vi "serialization tests.vi"() -> ()   [LabVIEW 2013, in "Modbus Slave tests.lvlib"]
doc: "Platypus Framework 1.0.1.65\nNI Systems Engineering - National Instruments"
uses:
  Modbus Slave tests.lvlib
  configuration/Modbus Slave configuration.lvclass
  configuration/Modbus Slave configuration.lvclass/Modbus Slave configuration.ctl
  configuration/Read modbus channels.vi
  configuration/Read port (502).vi
panel:
  out "ok":bool
  out "no error":errorcluster
  out "no error":errorcluster
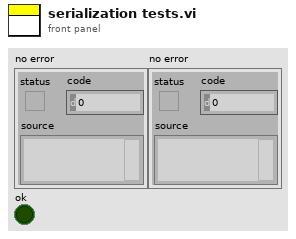
[diagram p1: front panel]
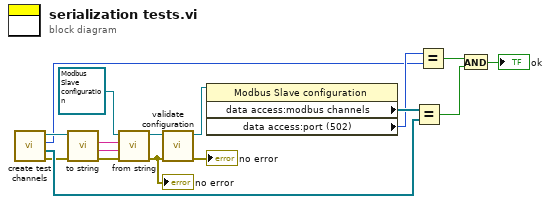
[diagram p0: block diagram]
diagram:
  n1 = call "create test channels.vi"() -> ("error out"=w8:errorcluster, "Array"=w9:refnum<class "Modbus Module Channel.lvclass">[], "port (502)"=w3:u16, "Modbus Slave configuration out"=w10:refnum<class "Modbus Slave configuration.lvclass">)  [unwired: 7 in, 1 out]
  n2 = call-dynamic "to string.vi"("error in"=w8, "Modbus Slave configuration in"=w10) -> ("error out"=w17:errorcluster, "data"=w16:string, "version"=w15:string)  [unwired: 6 in, 1 out]
  n3 = call-dynamic "from string.vi"("error in"=w17, "data"=w16, "version"=w15, "Modbus Slave configuration in"=refnum<class "Modbus Slave configuration.lvclass"> refnum ("tag bus configurable plugin module configuration")) -> ("error out"=w12:errorcluster, "Modbus Slave configuration out"=w14:refnum<class "Modbus Slave configuration.lvclass">)  [unwired: 6 in]
  "no error" <- w12
  n4 = call-dynamic "validate configuration.vi"("error in"=w12, "Modbus Slave configuration in"=w14) -> ("error out"=→"no error":errorcluster, "Modbus Slave configuration out"=w6:refnum<class "Modbus Slave configuration.lvclass">)  [unwired: 8 in]
  n5 = property class="Modbus Slave configuration"(reference=w6) -> ("data access:modbus channels"=w5:refnum<class "Modbus Module Channel.lvclass">[], "data access:port (502)"=w4:u16)  [unwired: 1 in, 2 out]
  n6 = Equal?(x=w5, y=w9) -> (x = y?=w11:bool)
  n7 = Equal?(x=w4, y=w3) -> (x = y?=w1:bool)
  n8 = And(x=w1, y=w11) -> (x .and. y?=→"ok":bool)
